vi "Write AttackerAngleToShootInDegrees.vi"(8 "error in (no error)":errorcluster, 10 "AttackerAngle\nToTurnInDegrees":dbl, 11 "Parameters in":refnum<class "Parameters.lvclass">) -> (0 "error out":errorcluster, 3 "Parameters out":refnum<class "Parameters.lvclass">)   [LabVIEW 2020, in "Parameters.lvclass"]
uses:
  Parameters.lvclass
  Parameters.lvclass/Parameters.ctl
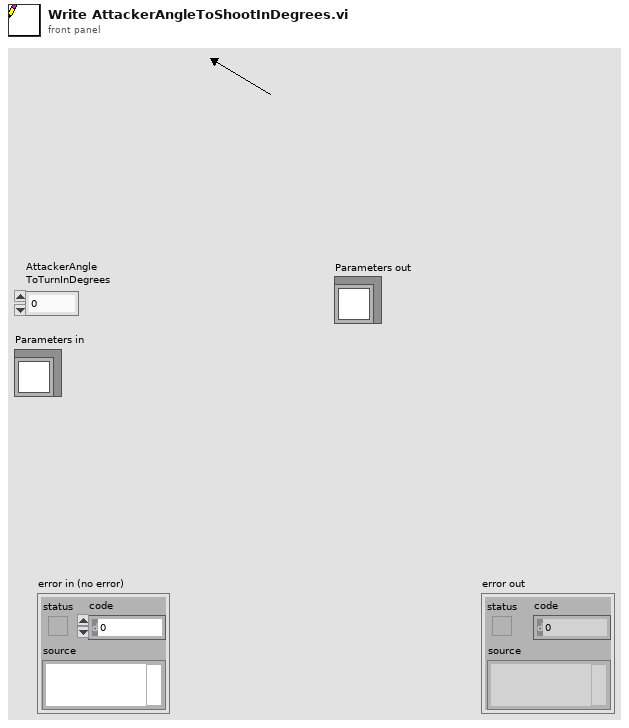
[diagram p1: front panel]
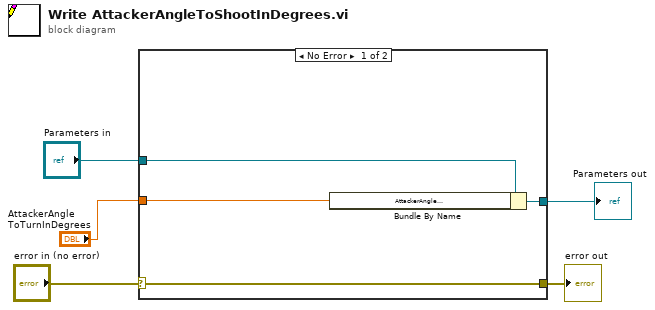
[diagram p0: block diagram]
diagram:
  n1 = case shown="No Error" "error in (no error)" {
    selector: "error in (no error)" -> [w9 w11]
    tunnel: [w9 w11] -> w4
    tunnel: [w8 w10] -> w2
    tunnel: "Parameters in" -> [w7 w10]
    tunnel: "AttackerAngle\nToTurnInDegrees" -> [w6 _]
    frame No Error {
      n2 = Bundle By Name(cluster=w7, "AttackerAngle\nToShootInDegrees"=w6) -> (w8:refnum<class "Parameters.lvclass">)
    }
    frame Error {
    }
  }
  "error out" <- w4
  "Parameters out" <- w2
